vi "S2C_M2p5942_Proc_GetData.vi"(7 "Command":string, 8 "Error In":errorcluster, 10 "Ready?":bool, 11 "Card In":cluster{"Card Handle":u64, "Error Code":u32}) -> (0 "Error Out":errorcluster, 3 "Card Out":cluster{"Card Handle":u64, "Error Code":u32})   [LabVIEW 2024]
uses:
  S2C_M2p5942_Proc_Globals.vi
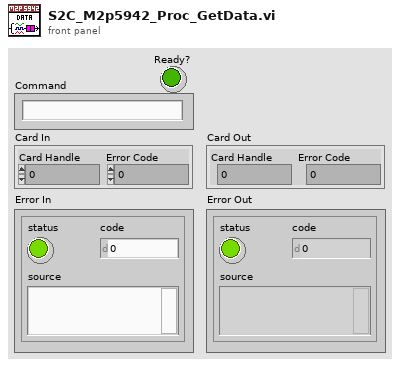
[diagram p1: front panel]
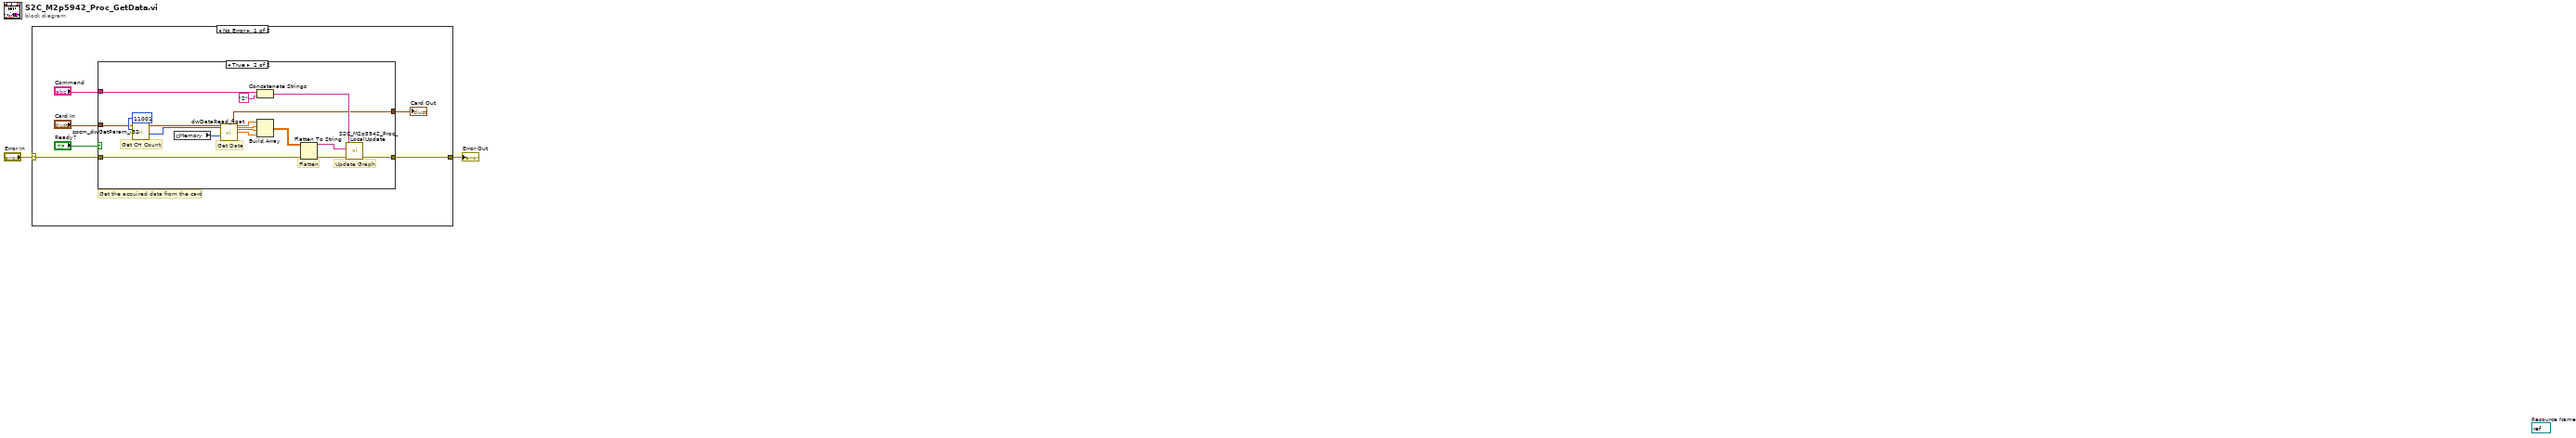
[diagram p0: block diagram]
diagram:
  (unwired) refnum<visa-resource-name> refnum  # Resource Name
  n1 = case shown="No Error" "Error In" {
    selector: "Error In" -> [w8 w29]
    tunnel: [w5 w29] -> w1
    frame No Error {
      # "Get the acquired data from the card"
      n2 = case shown="True" "Ready?" {
        tunnel: w8 -> [w10 w20]
        tunnel: "Card In" -> [w9 w27]
        tunnel: "Command" -> [_ w16]
        tunnel: [w10 w13] -> w5
        tunnel: [w9 w12] -> w3
        frame False {
        }
        frame True {
          # "Get Data"
          # "Get CH Count"
          # "Flatten"
          # "Update Graph"
          n3 = call "spcm_dwGetParam_i32.vi"("Register"=11001, "Card Info In"=w27) -> ("Value (int32)"=w25:i32, "Card Info Out"=w26:cluster{"Card Handle":u64, "Error Code":u32})  [unwired: 4 in]
          n4 = global read "S2C_M2p5942_Proc_Globals.vi" "Memory"() -> (w11:u32)
          n5 = call "dwDataRead_float.vi"("Card Info In"=w26, "Channel Count"=w25, "Length (Samples per Channel)"=w11) -> ("Card Info Out"=w12:cluster{"Card Handle":u64, "Error Code":u32}, "Ch 0"=w24:sgl[], "Ch 1"=w23:sgl[], "Ch 2"=w22:sgl[], "Ch 3"=w21:sgl[])  [unwired: 8 in, 12 out]
          n6 = Concatenate Strings(w16, "2" ("string")) -> (w15:string)
          n7 = Build Array(w24, w23, w22, w21) -> (w19:sgl[][])
          n8 = Flatten To String(anything=w19, error in (no error)=w20) -> (data string=w14:string, error out=w18:errorcluster)  [unwired: 2 in, 1 out]
          n9 = call "S2C_M2p5942_Proc_LocalUpdate.vi"("Error In"=w18, "Data"=w14, "Command"=w15) -> ("Error Out"=w13:errorcluster)  [unwired: 8 in]
        }
      }
      "Card Out" <- w3
    }
    frame Error {
    }
  }
  "Error Out" <- w1
